vi "CRYMenu Language Set.vi"(10 "sID":string) -> (0 "sShortcut_Out":string, 1 "sMultibyte_Out":string, 2 "sID_Out":string, 3 "sUnicode_Out":string)   [LabVIEW 2013]
uses:
  CRYMainGlobal.vi
panel:
  in  "sIDUnicode":string
  # "MultiLanguage Menu String Array"
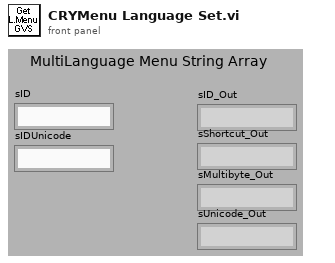
[diagram p1: front panel]
types:
  T1 = enum32{"English", "Chinese", "Korean", "Japanese", "Russian", "Chinese traditional"}
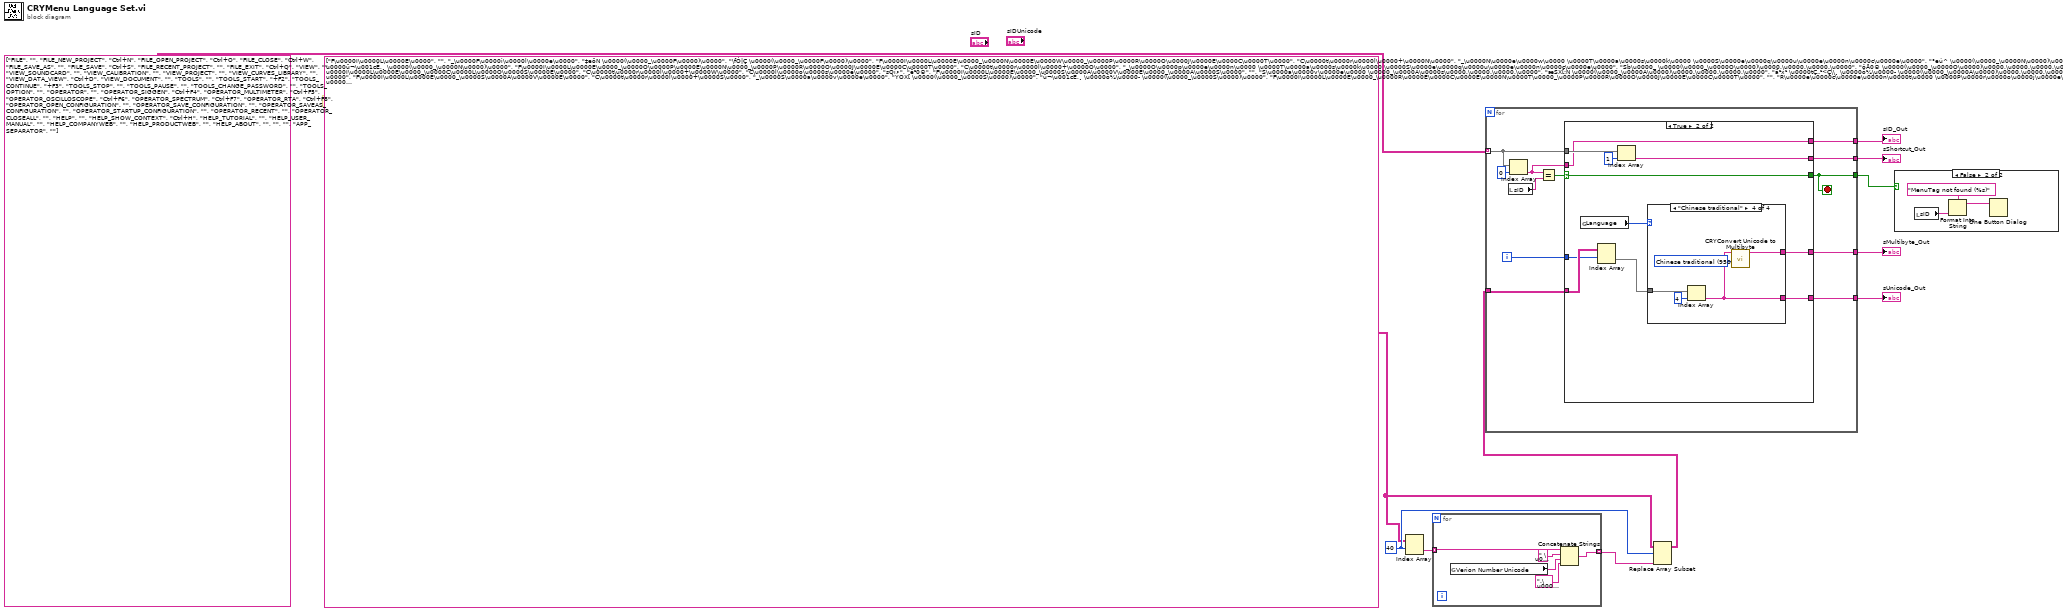
[diagram p0: block diagram]
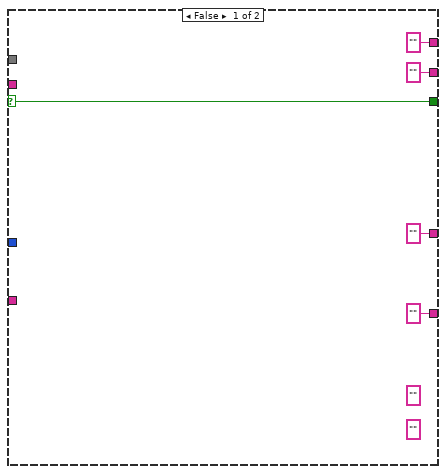
[diagram p3: hidden frame]
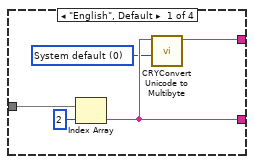
[diagram p4: hidden frame]
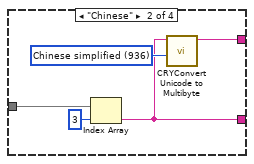
[diagram p5: hidden frame]
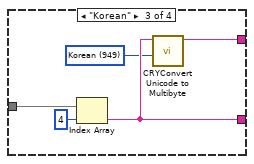
[diagram p6: hidden frame]
diagram:
  w4 = 40 ("disabled index (col)")
  w1 = string[][] [["F\u0000I\u0000L\u0000E\u0000", "", "_\u0000F\u0000i\u0000l\u0000e\u0000", "‡eöN \u0000(\u0000_\u0000F\u0000)\u0000", "\fÓ|Ç \u0000(\u0000_\u0000F\u0000)\u0000"], ["F\u0000I\u0000L\u0000E\u0000_\u0000N\u0000E\u0000W\u0000_\u0000P\u0000R\u0000O\u0000J\u0000E\u0000C\u0000T\u0000", "C\u0000t\u0000r\u0000l\u0000+\u0000N\u0000", "_\u0000N\u0000e\u0000w\u0000 \u0000T\u0000a\u0000s\u0000k\u0000 \u0000S\u0000e\u0000q\u0000u\u0000e\u0000n\u0000c\u0000e\u0000", "°eú^ \u0000(\u0000_\u0000N\u0000)\u0000", "ÈÀ \u0000ü¬\u001cÈ,¸ \u0000(\u0000_\u0000N\u0000)\u0000"], ["F\u0000I\u0000L\u0000E\u0000_\u0000O\u0000P\u0000E\u0000N\u0000_\u0000P\u0000R\u0000O\u0000J\u0000E\u0000C\u0000T\u0000", "C\u0000t\u0000r\u0000l\u0000+\u0000O\u0000", "_\u0000O\u0000p\u0000e\u0000n\u0000 \u0000T\u0000a\u0000s\u0000k\u0000 \u0000S\u0000e\u0000q\u0000u\u0000e\u0000n\u0000c\u0000e\u0000", "Sb\u0000_ \u0000(\u0000_\u0000O\u0000)\u0000.\u0000.\u0000.\u0000", "ôÅ0® \u0000(\u0000_\u0000O\u0000)\u0000.\u0000.\u0000.\u0000"], ["F\u0000I\u0000L\u0000E\u0000_\u0000C\u0000L\u0000O\u0000S\u0000E\u0000", "C\u0000t\u0000r\u0000l\u0000+\u0000W\u0000", "C\u0000l\u0000o\u0000s\u0000e\u0000", "sQí•", "ë²0®"], ["F\u0000I\u0000L\u0000E\u0000_\u0000S\u0000A\u0000V\u0000E\u0000_\u0000A\u0000S\u0000", "", "S\u0000a\u0000v\u0000e\u0000 \u0000_\u0000A\u0000s\u0000.\u0000.\u0000.\u0000", "æSX[:N \u0000(\u0000_\u0000A\u0000)\u0000.\u0000.\u0000.\u0000", "ä²x¹ \u0000tÇ„¹<Ç\\¸ \u0000ô¼\u0000­ \u0000(\u0000_\u0000A\u0000)\u0000.\u0000.\u0000.\u0000"], ["F\u0000I\u0000L\u0000E\u0000_\u0000S\u0000A\u0000V\u0000E\u0000", "C\u0000t\u0000r\u0000l\u0000+\u0000S\u0000", "_\u0000S\u0000a\u0000v\u0000e\u0000", "ÝOX[ \u0000(\u0000_\u0000S\u0000)\u0000", "ü¬\u001cÈ,¸ \u0000ô¼\u0000­ \u0000(\u0000_\u0000S\u0000)\u0000"], ["F\u0000I\u0000L\u0000E\u0000_\u0000R\u0000E\u0000C\u0000E\u0000N\u0000T\u0000_\u0000P\u0000R\u0000O\u0000J\u0000E\u0000C\u0000T\u0000", "", "R\u0000e\u0000c\u0000e\u0000n\u0000t\u0000 \u0000P\u0000r\u0000o\u0000j\u0000e\u0000c\u0000t\u0000s\u0000", "\u0000g°eSb\u0000_", "\\Íü­ \u0000¬¹©Æ\\Õ \u0000ü¬\u001cÈ,¸"], ["F\u0000I\u0000L\u0000E\u0000_\u0000E\u0000X\u0000I\u0000T\u0000", "C\u0000t\u0000r\u0000l\u0000+\u0000Q\u0000", "E\u0000_\u0000x\u0000i\u0000t\u0000", "\u0000úQ \u0000(\u0000_\u0000x\u0000)\u0000", "]°´°0® \u0000(\u0000_\u0000x\u0000)\u0000"], ["V\u0000I\u0000E\u0000W\u0000", "", "_\u0000V\u0000i\u0000e\u0000w\u0000", "Omȉ \u0000(\u0000_\u0000V\u0000)\u0000", "ô¼0® \u0000(\u0000_\u0000V\u0000)\u0000"], ["V\u0000I\u0000E\u0000W\u0000_\u0000S\u0000O\u0000U\u0000N\u0000D\u0000C\u0000A\u0000R\u0000D\u0000", "", "S\u0000o\u0000u\u0000n\u0000d\u0000C\u0000a\u0000r\u0000d\u0000", "ðXaS", "LÇ1ÁtÎÜ´"], ["V\u0000I\u0000E\u0000W\u0000_\u0000C\u0000A\u0000L\u0000I\u0000B\u0000R\u0000A\u0000T\u0000I\u0000O\u0000N\u0000", "", "C\u0000a\u0000l\u0000i\u0000b\u0000r\u0000a\u0000t\u0000i\u0000o\u0000n\u0000", "!hÆQ", "P­\u0000É"], ["V\u0000I\u0000E\u0000W\u0000_\u0000P\u0000R\u0000O\u0000J\u0000E\u0000C\u0000T\u0000", "", "_\u0000P\u0000r\u0000o\u0000j\u0000e\u0000c\u0000t\u0000", "^\u0017R \u0000(\u0000_\u0000P\u0000)\u0000", "ü¬\u001cÈ,¸¸ÓÑÉ0®=Ì8» \u0000(\u0000_\u0000P\u0000)\u0000"], ["V\u0000I\u0000E\u0000W\u0000_\u0000C\u0000U\u0000R\u0000V\u0000E\u0000S\u0000_\u0000L\u0000I\u0000B\u0000R\u0000A\u0000R\u0000Y\u0000", "", "_\u0000C\u0000u\u0000r\u0000v\u0000e\u0000s\u0000 \u0000L\u0000i\u0000b\u0000r\u0000a\u0000r\u0000y\u0000", "òf¿~“^ \u0000(\u0000_\u0000C\u0000)\u0000", "á¬ Á\u001cÁà¬=Ì8» \u0000(\u0000_\u0000C\u0000)\u0000"], ["V\u0000I\u0000E\u0000W\u0000_\u0000D\u0000A\u0000T\u0000A\u0000_\u0000V\u0000I\u0000E\u0000W\u0000", "C\u0000t\u0000r\u0000l\u0000+\u0000D\u0000", "_\u0000D\u0000a\u0000t\u0000a\u0000 \u0000V\u0000i\u0000e\u0000w\u0000", "þVhˆ \u0000(\u0000_\u0000D\u0000)\u0000", "ÇÌ¸ô¼0®=Ì8» \u0000(\u0000_\u0000D\u0000)\u0000"], ["V\u0000I\u0000E\u0000W\u0000_\u0000D\u0000O\u0000C\u0000U\u0000M\u0000E\u0000N\u0000T\u0000", "", "D\u0000o\u0000c\u0000u\u0000_\u0000m\u0000e\u0000n\u0000t\u0000", "¥bhˆ \u0000(\u0000_\u0000m\u0000)\u0000", "8»\u001cÁ¸ÓÑÉ=Ì8» \u0000(\u0000_\u0000m\u0000)\u0000"], ["T\u0000O\u0000O\u0000L\u0000S\u0000", "", "_\u0000T\u0000o\u0000o\u0000l\u0000s\u0000", "\ty \u0000(\u0000_\u0000T\u0000)\u0000", "ü¬\u001cÈ,¸ \u0000pÈ…È \u0000(\u0000_\u0000T\u0000)\u0000"], ["T\u0000O\u0000O\u0000L\u0000S\u0000_\u0000S\u0000T\u0000A\u0000R\u0000T\u0000", "+\u0000F\u00002\u0000", "_\u0000S\u0000t\u0000a\u0000r\u0000t\u0000", "\u0000_ËY \u0000(\u0000_\u0000S\u0000)\u0000", "äÂ‰Õ \u0000(\u0000_\u0000S\u0000)\u0000"], ["T\u0000O\u0000O\u0000L\u0000S\u0000_\u0000C\u0000O\u0000N\u0000T\u0000I\u0000N\u0000U\u0000E\u0000", "+\u0000F\u00003\u0000", "_\u0000C\u0000o\u0000n\u0000t\u0000i\u0000n\u0000u\u0000e\u0000", "ç~í~ \u0000(\u0000_\u0000C\u0000)\u0000", "(¸ÁäÂÕ \u0000(\u0000_\u0000C\u0000)\u0000"], ["T\u0000O\u0000O\u0000L\u0000S\u0000_\u0000S\u0000T\u0000O\u0000P\u0000", "", "S\u0000_\u0000t\u0000o\u0000p\u0000", "-N­e \u0000(\u0000_\u0000t\u0000)\u0000", "äÂ‰Õ\u0011ÉÀÉ \u0000(\u0000_\u0000t\u0000)\u0000"], ["T\u0000O\u0000O\u0000L\u0000S\u0000_\u0000P\u0000A\u0000U\u0000S\u0000E\u0000", "", "_\u0000P\u0000a\u0000u\u0000s\u0000e\u0000", "‚f\\P \u0000(\u0000_\u0000P\u0000)\u0000", "¼¹ÜÂ\u0011ÉÀÉ \u0000(\u0000_\u0000P\u0000)\u0000"], ["T\u0000O\u0000O\u0000L\u0000S\u0000_\u0000C\u0000H\u0000A\u0000N\u0000G\u0000E\u0000_\u0000P\u0000A\u0000S\u0000S\u0000W\u0000O\u0000R\u0000D\u0000", "", "_\u0000L\u0000o\u0000g\u0000i\u0000n\u0000.\u0000.\u0000.\u0000", "{vU_ \u0000(\u0000_\u0000R\u0000)\u0000.\u0000.\u0000.\u0000", "ñ´]¸ \u0000(\u0000_\u0000R\u0000)\u0000.\u0000.\u0000.\u0000"], ["T\u0000O\u0000O\u0000L\u0000S\u0000_\u0000O\u0000P\u0000T\u0000I\u0000O\u0000N\u0000", "", "_\u0000O\u0000p\u0000t\u0000i\u0000o\u0000n\u0000.\u0000.\u0000.\u0000", "\ty \u0000(\u0000_\u0000O\u0000)\u0000.\u0000.\u0000.\u0000", "XÖ½¬$Á\u0015È \u0000(\u0000_\u0000O\u0000)\u0000.\u0000.\u0000.\u0000"], ["O\u0000P\u0000E\u0000R\u0000A\u0000T\u0000O\u0000R\u0000", "", "_\u0000O\u0000p\u0000e\u0000r\u0000a\u0000t\u0000o\u0000r\u0000", "Íd\\O \u0000(\u0000_\u0000O\u0000)\u0000", "äÂÜÂ\u0004¬ü¬\u001cÈ \u0000(\u0000_\u0000O\u0000)\u0000"], ["O\u0000P\u0000E\u0000R\u0000A\u0000T\u0000O\u0000R\u0000_\u0000S\u0000I\u0000G\u0000G\u0000E\u0000N\u0000", "", "S\u0000i\u0000g\u0000n\u0000a\u0000l\u0000 \u0000_\u0000G\u0000e\u0000n\u0000e\u0000r\u0000a\u0000t\u0000o\u0000r\u0000.\u0000.\u0000.\u0000", "áO÷SÑS\u001fuhV \u0000(\u0000_\u0000G\u0000)\u0000.\u0000.\u0000.\u0000", "àÂ8Ö\u001c¼ÝÀ0® \u0000(\u0000_\u0000G\u0000)\u0000.\u0000.\u0000.\u0000"], ["O\u0000P\u0000E\u0000R\u0000A\u0000T\u0000O\u0000R\u0000_\u0000M\u0000U\u0000L\u0000T\u0000I\u0000M\u0000E\u0000T\u0000E\u0000R\u0000", "", "_\u0000M\u0000u\u0000l\u0000t\u0000i\u0000m\u0000e\u0000t\u0000e\u0000r\u0000.\u0000.\u0000.\u0000", "\u0007N(uhˆ \u0000(\u0000_\u0000M\u0000)\u0000.\u0000.\u0000.\u0000", "Ì¹¥²!Î\u0015ÈÄ¬0® \u0000(\u0000_\u0000M\u0000)\u0000.\u0000.\u0000.\u0000"], ["O\u0000P\u0000E\u0000R\u0000A\u0000T\u0000O\u0000R\u0000_\u0000O\u0000S\u0000C\u0000I\u0000L\u0000L\u0000O\u0000S\u0000C\u0000O\u0000P\u0000E\u0000", "", "_\u0000O\u0000s\u0000c\u0000i\u0000l\u0000l\u0000o\u0000s\u0000c\u0000o\u0000p\u0000e\u0000.\u0000.\u0000.\u0000", ":yâlhV \u0000(\u0000_\u0000O\u0000)\u0000.\u0000.\u0000.\u0000", "$Æ0Å\\¸¤ÂTÏ\u0004Õ \u0000(\u0000_\u0000O\u0000)\u0000.\u0000.\u0000.\u0000"], ["O\u0000P\u0000E\u0000R\u0000A\u0000T\u0000O\u0000R\u0000_\u0000S\u0000P\u0000E\u0000C\u0000T\u0000R\u0000U\u0000M\u0000", "", "S\u0000_\u0000p\u0000e\u0000c\u0000t\u0000r\u0000u\u0000m\u0000 \u0000A\u0000n\u0000a\u0000l\u0000y\u0000z\u0000e\u0000r\u0000.\u0000.\u0000.\u0000", "1\u0006RghV \u0000(\u0000_\u0000p\u0000)\u0000.\u0000.\u0000.\u0000", "¤Â™Ó¸Òt¹„½\u001dÁ0® \u0000(\u0000_\u0000p\u0000)\u0000.\u0000.\u0000.\u0000"], ["O\u0000P\u0000E\u0000R\u0000A\u0000T\u0000O\u0000R\u0000_\u0000R\u0000T\u0000A\u0000", "", "_\u0000R\u0000e\u0000a\u0000l\u0000T\u0000i\u0000m\u0000e\u0000 \u0000A\u0000n\u0000a\u0000l\u0000y\u0000z\u0000e\u0000r\u0000.\u0000.\u0000.\u0000", "\rP\u000bz\u0006RghV \u0000(\u0000_\u0000R\u0000)\u0000.\u0000.\u0000.\u0000", "%ÆÀÐ\f¾„½\u001dÁ0® \u0000(\u0000_\u0000R\u0000)\u0000.\u0000.\u0000.\u0000"], ["O\u0000P\u0000E\u0000R\u0000A\u0000T\u0000O\u0000R\u0000_\u0000O\u0000P\u0000E\u0000N\u0000_\u0000C\u0000O\u0000N\u0000F\u0000I\u0000G\u0000U\u0000R\u0000A\u0000T\u0000I\u0000O\u0000N\u0000", "", "O\u0000p\u0000e\u0000n\u0000 \u0000_\u0000C\u0000o\u0000n\u0000f\u0000i\u0000g\u0000u\u0000r\u0000a\u0000t\u0000i\u0000o\u0000n\u0000.\u0000.\u0000.\u0000", "Sb\u0000_M‘n \u0000(\u0000_\u0000C\u0000)\u0000.\u0000.\u0000.\u0000", "XÖ½¬\fÓ|Ç \u0000ôÅ0® \u0000(\u0000_\u0000C\u0000)\u0000.\u0000.\u0000.\u0000"], ["O\u0000P\u0000E\u0000R\u0000A\u0000T\u0000O\u0000R\u0000_\u0000S\u0000A\u0000V\u0000E\u0000_\u0000C\u0000O\u0000N\u0000F\u0000I\u0000G\u0000U\u0000R\u0000A\u0000T\u0000I\u0000O\u0000N\u0000", "", "_\u0000S\u0000a\u0000v\u0000e\u0000 \u0000C\u0000o\u0000n\u0000f\u0000i\u0000g\u0000u\u0000r\u0000a\u0000t\u0000i\u0000o\u0000n\u0000", "ÝOX[M‘n \u0000(\u0000_\u0000S\u0000)\u0000", "XÖ½¬\fÓ|Ç \u0000ô¼\u0000­ \u0000(\u0000_\u0000S\u0000)\u0000"], ["O\u0000P\u0000E\u0000R\u0000A\u0000T\u0000O\u0000R\u0000_\u0000S\u0000A\u0000V\u0000E\u0000_\u0000C\u0000O\u0000N\u0000F\u0000I\u0000G\u0000U\u0000R\u0000A\u0000T\u0000I\u0000O\u0000N\u0000A\u0000S\u0000", "", "S\u0000a\u0000v\u0000e\u0000 \u0000C\u0000o\u0000n\u0000f\u0000i\u0000g\u0000u\u0000r\u0000a\u0000t\u0000i\u0000o\u0000n\u0000 \u0000_\u0000A\u0000s\u0000.\u0000.\u0000.\u0000", "æSX[M‘n:N \u0000(\u0000_\u0000A\u0000)\u0000.\u0000.\u0000.\u0000", "XÖ½¬\fÓ|Ç \u0000ä²x¹ \u0000tÇ„¹<Ç\\¸ \u0000ô¼\u0000­ \u0000(\u0000_\u0000A\u0000)\u0000.\u0000.\u0000.\u0000"], ["O\u0000P\u0000E\u0000R\u0000A\u0000T\u0000O\u0000R\u0000_\u0000S\u0000T\u0000A\u0000R\u0000T\u0000U\u0000P\u0000_\u0000C\u0000O\u0000N\u0000F\u0000I\u0000G\u0000U\u0000R\u0000A\u0000T\u0000I\u0000O\u0000N\u0000", "", "S\u0000t\u0000a\u0000r\u0000t\u0000u\u0000p\u0000 \u0000C\u0000o\u0000n\u0000f\u0000i\u0000g\u0000u\u0000r\u0000a\u0000t\u0000i\u0000o\u0000n\u0000.\u0000.\u0000.\u0000", "Øž¤‹M‘n.\u0000.\u0000.\u0000", "ÜÂ‘ÇXÖ½¬\fÓ|Ç \u0000 ÁÝÐ.\u0000.\u0000.\u0000"], ["O\u0000P\u0000E\u0000R\u0000A\u0000T\u0000O\u0000R\u0000_\u0000R\u0000E\u0000C\u0000E\u0000N\u0000T\u0000", "", "R\u0000e\u0000c\u0000e\u0000n\u0000t\u0000l\u0000y\u0000 \u0000O\u0000p\u0000e\u0000n\u0000e\u0000d\u0000 \u0000C\u0000o\u0000n\u0000f\u0000i\u0000g\u0000u\u0000r\u0000a\u0000t\u0000i\u0000o\u0000n\u0000s\u0000", "\u0000gя", "\\Íü­ \u0000¬¹©Æ\\Õ \u0000XÖ½¬\fÓ|Ç"], ["O\u0000P\u0000E\u0000R\u0000A\u0000T\u0000O\u0000R\u0000_\u0000C\u0000L\u0000O\u0000S\u0000E\u0000A\u0000L\u0000L\u0000", "", "C\u0000l\u0000o\u0000s\u0000e\u0000 \u0000A\u0000l\u0000l\u0000", "hQèsQí", "¨ºà´ \u0000=Ì8»ë²0®"], ["H\u0000E\u0000L\u0000P\u0000", "", "_\u0000H\u0000e\u0000l\u0000p\u0000", ".^©R \u0000(\u0000_\u0000H\u0000)\u0000", ")¼pÈ \u0000(\u0000_\u0000H\u0000)\u0000"], ["H\u0000E\u0000L\u0000P\u0000_\u0000S\u0000H\u0000O\u0000W\u0000_\u0000C\u0000O\u0000N\u0000T\u0000E\u0000X\u0000T\u0000", "C\u0000t\u0000r\u0000l\u0000+\u0000H\u0000", "_\u0000S\u0000h\u0000o\u0000w\u0000 \u0000C\u0000o\u0000n\u0000t\u0000e\u0000x\u0000t\u0000 \u0000H\u0000e\u0000l\u0000p\u0000", ">f:y\nN\u000bN‡e.^©R \u0000(\u0000_\u0000S\u0000)\u0000", "$ÁXÎ$Á…º\u001cÁ \u0000(\u0000_\u0000S\u0000)\u0000"], ["H\u0000E\u0000L\u0000P\u0000_\u0000T\u0000U\u0000T\u0000O\u0000R\u0000I\u0000A\u0000L\u0000", "", "_\u0000T\u0000u\u0000t\u0000o\u0000r\u0000i\u0000a\u0000l\u0000s\u0000", "ë_\u001f\nNKb\u0007cWS \u0000(\u0000_\u0000T\u0000)\u0000", "\bÍYÕÇ|¹ \u0000\u0004Ç\\Õ \u0000$Áº\u001cÁ \u0000(\u0000_\u0000T\u0000)\u0000"], ["H\u0000E\u0000L\u0000P\u0000_\u0000U\u0000S\u0000E\u0000R\u0000_\u0000M\u0000A\u0000N\u0000U\u0000A\u0000L\u0000", "", "U\u0000s\u0000e\u0000r\u0000 \u0000_\u0000M\u0000a\u0000n\u0000u\u0000a\u0000l\u0000", "(u7bKbŒQ \u0000(\u0000_\u0000M\u0000)\u0000", "¬À©Æ$Á…º\u001cÁ \u0000(\u0000_\u0000M\u0000)\u0000"], ["H\u0000E\u0000L\u0000P\u0000_\u0000C\u0000O\u0000M\u0000P\u0000A\u0000N\u0000Y\u0000W\u0000E\u0000B\u0000", "", "C\u0000R\u0000Y\u0000 \u0000S\u0000o\u0000u\u0000n\u0000d\u0000 \u0000C\u0000o\u0000.\u0000,\u0000 \u0000L\u0000t\u0000d\u0000.\u0000 \u0000W\u0000e\u0000b\u0000s\u0000i\u0000t\u0000e\u0000", "mgÞ]FQNS5uP[\tgP–lQøSQÙz \u0000(\u0000_\u0000W\u0000)\u0000", "\u001c¬\u001c¼½¬%¸ \u0000(\u0000_\u0000W\u0000)\u0000"], ["H\u0000E\u0000L\u0000P\u0000_\u0000P\u0000R\u0000O\u0000D\u0000U\u0000C\u0000T\u0000W\u0000E\u0000B\u0000", "", "C\u0000R\u0000Y\u0000 \u0000S\u0000o\u0000u\u0000n\u0000d\u0000 \u0000C\u0000o\u0000.\u0000,\u0000 \u0000L\u0000t\u0000d\u0000.\u0000 \u0000P\u0000r\u0000o\u0000d\u0000u\u0000c\u0000t\u0000i\u0000o\u0000n\u0000", "§NÁTáOo` \u0000(\u0000_\u0000P\u0000)\u0000", "\u001cÈˆÔ\u0015Èô¼ \u0000(\u0000_\u0000P\u0000)\u0000"], ["H\u0000E\u0000L\u0000P\u0000_\u0000A\u0000B\u0000O\u0000U\u0000T\u0000", "", "_\u0000A\u0000b\u0000o\u0000u\u0000t\u0000 \u0000C\u0000R\u0000Y\u00006\u00001\u00008\u00001\u0000 \u0000E\u0000l\u0000e\u0000c\u0000t\u0000r\u0000o\u0000-\u0000a\u0000c\u0000o\u0000u\u0000s\u0000t\u0000i\u0000c\u0000 \u0000A\u0000n\u0000a\u0000l\u0000y\u0000s\u0000i\u0000s\u0000 \u0000S\u0000y\u0000s\u0000t\u0000e\u0000m\u0000", "sQN \u0000C\u0000R\u0000Y\u00006\u00001\u00008\u00001\u0000 \u00005uðX\u0006Rgû|ß~", "LÇ¥ÕtÕ\u001dÁ\u0004Õ\\¸ø­Œ·ÐÅ \u0000\u0000³XÕìÅ"], ["", "", "", "", ""], ["A\u0000P\u0000P\u0000_\u0000S\u0000E\u0000P\u0000A\u0000R\u0000A\u0000T\u0000O\u0000R\u0000", "", "-\u0000", "-\u0000", "-\u0000"]]
  # "ASCIICODE"
  # "ID UNICODE(no Use)"
  n1 = Index Array(array=w1, index (row)=w4) -> (element=w5:string[])  [unwired: 1 in]
  n2 = for {
    tunnel: w5 -> [w16] mode=indexing
    tunnel: [w15] -> w3 mode=indexing
    n3 = global read "CRYMainGlobal.vi" "Verion Number Unicode"() -> (w14:string)
    n4 = Concatenate Strings(w16, " \u0000" ("message"), w14, ".\u0000.\u0000.\u0000" ("message")) -> (w15:string)
  }
  n5 = Replace Array Subset(array=w1, new element=w3, index (row)=w4) -> (w2:string[][])  [unwired: 1 in]
  n6 = for {
    tunnel: w2 -> [w27]
    tunnel: [w25] -> w11
    tunnel: [w24] -> w10
    tunnel: string[][] [["FILE", ""], ["FILE_NEW_PROJECT", "Ctrl+N"], ["FILE_OPEN_PROJECT", "Ctrl+O"], ["FILE_CLOSE", "Ctrl+W"], ["FILE_SAVE_AS", ""], ["FILE_SAVE", "Ctrl+S"], ["FILE_RECENT_PROJECT", ""], ["FILE_EXIT", "Ctrl+Q"], ["VIEW", ""], ["VIEW_SOUNDCARD", ""], ["VIEW_CALIBRATION", ""], ["VIEW_PROJECT", ""], ["VIEW_CURVES_LIBRARY", ""], ["VIEW_DATA_VIEW", "Ctrl+D"], ["VIEW_DOCUMENT", ""], ["TOOLS", ""], ["TOOLS_START", "+F2"], ["TOOLS_CONTINUE", "+F3"], ["TOOLS_STOP", ""], ["TOOLS_PAUSE", ""], ["TOOLS_CHANGE_PASSWORD", ""], ["TOOLS_OPTION", ""], ["OPERATOR", ""], ["OPERATOR_SIGGEN", "Ctrl+F4"], ["OPERATOR_MULTIMETER", "Ctrl+F5"], ["OPERATOR_OSCILLOSCOPE", "Ctrl+F6"], ["OPERATOR_SPECTRUM", "Ctrl+F7"], ["OPERATOR_RTA", "Ctrl+F8"], ["OPERATOR_OPEN_CONFIGURATION", ""], ["OPERATOR_SAVE_CONFIGURATION", ""], ["OPERATOR_SAVEAS_CONFIGURATION", ""], ["OPERATOR_STARTUP_CONFIGURATION", ""], ["OPERATOR_RECENT", ""], ["OPERATOR_CLOSEALL", ""], ["HELP", ""], ["HELP_SHOW_CONTEXT", "Ctrl+H"], ["HELP_TUTORIAL", ""], ["HELP_USER_MANUAL", ""], ["HELP_COMPANYWEB", ""], ["HELP_PRODUCTWEB", ""], ["HELP_ABOUT", ""], ["", ""], ["APP_SEPARATOR", ""]] -> [w21] mode=indexing
    tunnel: [w20] -> w7
    tunnel: [w18] -> w8
    tunnel: [w17] -> w6
    i -> [w23]
    stop <- w17 stop-if-true
    n7 = local read "sID"() -> (w28:string)
    n8 = Index Array(array=w21, index=0) -> (element=w19:string)
    n9 = Equal?(x=w19, y=w28) -> (x = y?=w26:bool)
    n10 = case shown="True" w26 {
      selector: w26 -> [w31 w42]
      tunnel: w27 -> [_ w41]
      tunnel: ["" ("Multibyte string") w44] -> w25
      tunnel: ["" w43] -> w24
      tunnel: [w31 w42] -> w17
      tunnel: w23 -> [_ w40]
      tunnel: w21 -> [_ w37]
      tunnel: ["" w36] -> w20
      tunnel: w19 -> [_ w35]
      tunnel: ["" w35] -> w18
      frame False {
        (unwired) ""
        (unwired) ""
      }
      frame True {
        n11 = global read "CRYMainGlobal.vi" "Language"() -> (w34:T1)
        n12 = Index Array(array=w41, index (row)=w40) -> (element=w39:string[])  [unwired: 1 in]
        n13 = Index Array(array=w37, index=1) -> (element=w36:string)
        n14 = case shown="\"Chinese traditional\"" w34 {
          tunnel: w39 -> [w49 w52 w56 w61]
          tunnel: [w47 w50 w57 w62] -> w43
          tunnel: [w45 w51 w58 w63] -> w44
          frame "English", Default {
            w46 = 0 items=["System default"=0, "Latin-1"=1252, "Japanese"=932, "Korean"=947, "Chinese simplified"=936, "Chinese traditional"=950, "Central Europe"=1250, "Cyrillic"=1251, "Greek"=1253, "Turkish"=1254, "Hebrew"=1255, "Arabic"=1256, "Baltic"=1257, "Thai"=874, "Vietnamese"=783, "UTF8"=65001, "UTF-7"=65000] ("Code Page")
            n15 = Index Array(array=w49, index=2) -> (element=w47:string)
            n16 = call "CRYConvert Unicode to Multibyte.vi"("Code Page"=w46, "Unicode String"=w47) -> ("Multibyte string"=w45:string)  [unwired: 8 in, 1 out]
          }
          frame "Chinese" {
            w53 = 936 items=["System default"=0, "Latin-1"=1252, "Japanese"=932, "Korean"=947, "Chinese simplified"=936, "Chinese traditional"=950, "Central Europe"=1250, "Cyrillic"=1251, "Greek"=1253, "Turkish"=1254, "Hebrew"=1255, "Arabic"=1256, "Baltic"=1257, "Thai"=874, "Vietnamese"=783, "UTF8"=65001, "UTF-7"=65000] ("Code Page")
            n17 = Index Array(array=w52, index=3) -> (element=w50:string)
            n18 = call "CRYConvert Unicode to Multibyte.vi"("Code Page"=w53, "Unicode String"=w50) -> ("Multibyte string"=w51:string)  [unwired: 8 in, 1 out]
          }
          frame "Korean" {
            w55 = 949 items=["System default"=0, "Latin-1"=1252, "Japanese"=932, "Korean"=949, "Chinese simplified"=936, "Chinese traditional"=950, "Central Europe"=1250, "Cyrillic"=1251, "Greek"=1253, "Turkish"=1254, "Hebrew"=1255, "Arabic"=1256, "Baltic"=1257, "Thai"=874, "Vietnamese"=783, "UTF8"=65001, "UTF-7"=65000] ("Code Page")
            n19 = Index Array(array=w56, index=4) -> (element=w57:string)
            n20 = call "CRYConvert Unicode to Multibyte.vi"("Code Page"=w55, "Unicode String"=w57) -> ("Multibyte string"=w58:string)  [unwired: 8 in, 1 out]
          }
          frame "Chinese traditional" {
            w60 = 950 items=["System default"=0, "Latin-1"=1252, "Japanese"=932, "Korean"=949, "Chinese simplified"=936, "Chinese traditional"=950, "Central Europe"=1250, "Cyrillic"=1251, "Greek"=1253, "Turkish"=1254, "Hebrew"=1255, "Arabic"=1256, "Baltic"=1257, "Thai"=874, "Vietnamese"=783, "UTF8"=65001, "UTF-7"=65000] ("Code Page")
            n21 = Index Array(array=w61, index=4) -> (element=w62:string)
            n22 = call "CRYConvert Unicode to Multibyte.vi"("Code Page"=w60, "Unicode String"=w62) -> ("Multibyte string"=w63:string)  [unwired: 8 in, 1 out]
          }
        }
      }
    }
  }
  "sMultibyte_Out" <- w11
  "sUnicode_Out" <- w10
  "sID_Out" <- w8
  "sShortcut_Out" <- w7
  n23 = case shown="False" w6 {
    frame True {
    }
    frame False {
      n24 = local read "sID"() -> (w66:string)
      n25 = Format Into String(format string="MenuTag not found (%s)", w66) -> (resulting string=w65:string)  [unwired: 2 in, 1 out]
      n26 = One Button Dialog(message=w65) -> ()  [unwired: 1 in, 1 out]
    }
  }
